vi "girada.vi"() -> ()   [LabVIEW 2021]
uses:
  Robot_class/Robot.lvclass
  Game_class/Game.lvclass
  Ally_class/Ally.lvclass
  Ball_class/Ball.lvclass
  Referee_class/Referee.lvclass
  Field_class/Field.lvclass
  Enemy_class/Enemy.lvclass
  Events_class/Events.lvclass
  Utilities_class/Utilities.lvclass
  Parameters_class/Parameters.lvclass
  Playbook_class/Playbook.lvclass
  Play_class/Play.lvclass
  TestPlay_class/TestPlay.lvclass
  EnemyPossessionAtEnemyFieldPlay_class/EnemyPossessionAtEnemyFieldPlay.lvclass
  EnemyPossessionAtOurFieldPlay_class/EnemyPossessionAtOurFieldPlay.lvclass
  NormalGamePlay_class/NormalGamePlay.lvclass
  IndirectEnemyPlay_class/IndirectEnemyPlay.lvclass
  PrepareKickoffAllyPlay_class/PrepareKickoffAllyPlay.lvclass
  PrepareKickoffEnemyPlay_class/PrepareKickoffEnemyPlay.lvclass
  KickPenaltyAllyPlay_class/KickPenaltyAllyPlay.lvclass
  PreparePenaltyAllyPlay_class/PreparePenaltyAllyPlay.lvclass
  DirectEnemyPlay_class/DirectEnemyPlay.lvclass
  PreparePenaltyEnemyPlay_class/PreparePenaltyEnemyPlay.lvclass
  BallOutOfFieldPlay_class/BallOutOfFieldPlay.lvclass
  StopOffensivePlay_class/StopOffensivePlay.lvclass
  PassPlay_class/PassPlay.lvclass
  DirectKickPlay_class/DirectKickPlay.lvclass
  HaltPlay_class/HaltPlay.lvclass
  PreparePassPlay_class/PreparePassPlay.lvclass
  PassToStriker_class/PassToStriker.lvclass
  PassTo2ndStriker_class/PassTo2ndStriker.lvclass
  SimplePass_class/SimplePass.lvclass
  PrepareRollToPassPlay_class/PrepareRollToPassPlay.lvclass
  PrepareDoublePassPlay_class/PrepareDoublePassPlay.lvclass
  TableWith2ndStrikerPlay_class/TableWith2ndStrikerPlay.lvclass
  TableWithStrikerPlay_class/TableWithStrikerPlay.lvclass
  PrepareTriplePassPlay_class/PrepareTriplePassPlay.lvclass
  ABCPassPlay_class/ABCPassPlay.lvclass
  PreparePassInGame1_class/PreparePassInGame1.lvclass
  ACBPassPlay_class/ACBPassPlay.lvclass
  PrepareKeeperPassPlay_class/PrepareKeeperPassPlay.lvclass
  KeeperPassToStrikerPlay_class/KeeperPassToStrikerPlay.lvclass
  5RobotsNormalGamePlay_class/5RobotsNormalGamePlay.lvclass
  Rolebook_class/Rolebook.lvclass
  5RobotsRole_class/5RobotsRole.lvclass
  Tacticbook_class/Tacticbook.lvclass
  ShootRole_class/ShootRole.lvclass
  5RobotsPassGamePlay_class/5RobotsPassGamePlay.lvclass
  PassBestRobotRole_class/PassBestRobotRole.lvclass
  PassBestReceiverRole_class/PassBestReceiverRole.lvclass
  5RobotsKeeperGame_class/5RobotsKeeperGame.lvclass
  5PreparePassGamePlay_class/5PreparePassGamePlay.lvclass
  NormalDefensivePlay_class/NormalDefensivePlay.lvclass
  NormalDefensiveWithDuelistPlay_class/NormalDefensiveWithDuelistPlay.lvclass
  KeeperPlay_class/KeeperPlay.lvclass
  KeeperRole_class/KeeperRole.lvclass
  TimeoutPlay_class/TimeoutPlay.lvclass
  ZigZagPlay_class/ZigZagPlay.lvclass
  GoToPlay_class/GoToPlay.lvclass
  BallPlacementPlay_class/BallPlacementPlay.lvclass
  BallPlacementAllyPlay_class/BallPlacementAllyPlay.lvclass
  SimpleBallPlacementAllyPlay_class/SimpleBallPlacementAllyPlay.lvclass
  RobotFeedback/RobotFeedback.lvclass
panel:
  out "String":string
  out "Robot out":refnum<class "Robot.lvclass">
  in  "Target":dbl[](array[numeric])
  in  "Robot in":refnum<class "Robot.lvclass">=refnum
  in  "Game in":refnum<class "Game.lvclass">=refnum
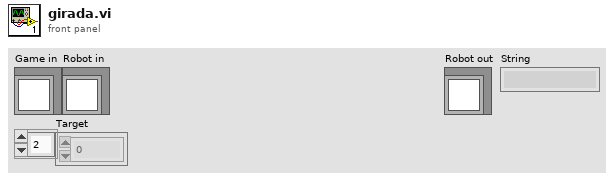
[diagram p1: front panel]
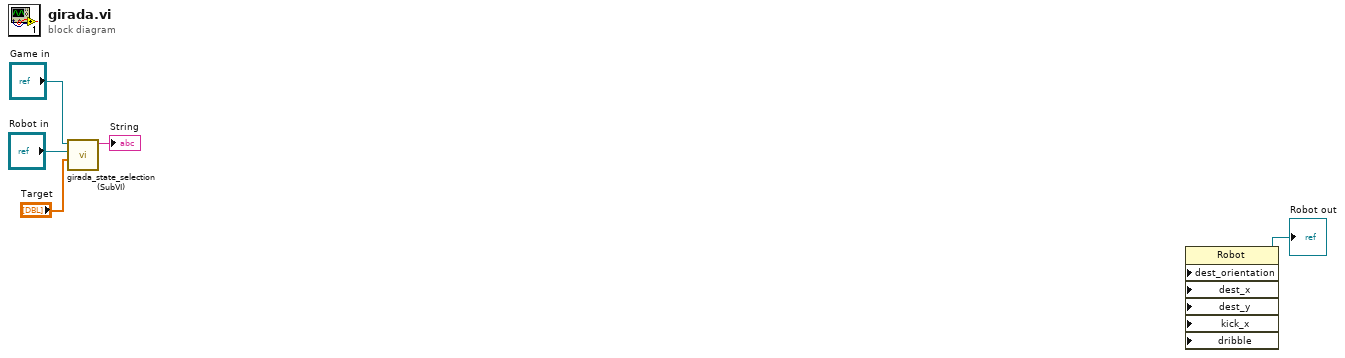
[diagram p0: block diagram]
diagram:
  n1 = call "girada_state_selection (SubVI).vi"("Target"="Target", "Robot in"="Robot in", "Game in"="Game in") -> ("String"=→"String":string)  [unwired: 8 in]
  n2 = property class="Robot" props=["dest_orientation", "dest_x", "dest_y", "kick_x", "dribble"]() -> (reference out=→"Robot out":refnum<class "Robot.lvclass">)  [unwired: 7 in, 1 out]
